vi "PH_SSAC.Translate Status.vi"(1 "Device Status":T1 items=["no info", "off/false/out", "on/true/in", "Failure", "Alarm", "Status 1", "Status 2", "Status 3"]) -> (0 "Translated Status":string)   [LabVIEW 2014, in "PH_SSAC.lvlib"]
doc: "This VI translates the device status in a human readable text."
uses:
  PH_SSAC.lvlib
  PH_Basics/PH_StatusHandler/PH_StatusHandler.Status.ctl
  PH_Basics/PH_StatusHandler/PH_StatusHandler.lvlib
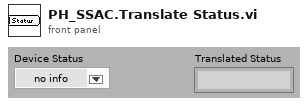
[diagram p1: front panel]
types:
  T1 = typedef "PH_StatusHandler.lvlib/PH_StatusHandler.Status.ctl" = i16
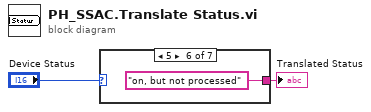
[diagram p0: block diagram]
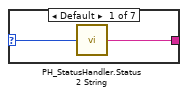
[diagram p2: hidden frame]
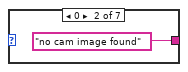
[diagram p3: hidden frame]
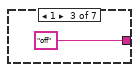
[diagram p4: hidden frame]
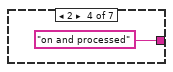
[diagram p5: hidden frame]
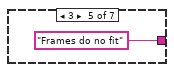
[diagram p6: hidden frame]
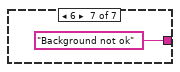
[diagram p7: hidden frame]
diagram:
  n1 = case shown="5" "Device Status" {
    selector: "Device Status" -> [w4 _ _ _ _ _ _]
    tunnel: [w3 "no cam image found" ("Device Status as string") "off" ("Device Status as string") "on and processed" ("Device Status as string") "Frames do no fit" ("Device Status as string") "on, but not processed" ("Device Status as string") "Background not ok" ("Device Status as string")] -> w1
    frame Default {
      n2 = call "PH_StatusHandler.Status 2 String.vi"("Status"=w4) -> ("Status as string"=w3:string)
    }
    frame 0 {
    }
    frame 1 {
    }
    frame 2 {
    }
    frame 3 {
    }
    frame 5 {
    }
    frame 6 {
    }
  }
  "Translated Status" <- w1
